vi "Sensors_DAQ.vi"() -> ()   [LabVIEW 2018]
uses:
  <vilib>/DAQmx/read.llb/DAQmx Read (Analog 1D Wfm NChan 1Samp).vi
  <vilib>/DAQmx/read.llb/DAQmx Read (Analog 1D Wfm NChan NSamp).vi
  <vilib>/DAQmx/miscellaneous.llb/DAQmx Fill In Error Info.vi
  Global.vi
panel:
  in  "Projects":string[](array[string])
  in  "Independent?":bool=TRUE
  out "file path 2":path=path "C:/Users/aspit/Git/MHDLab/Test Data/2018-06-02/H2TC/Temp Dependence/TestVI_Sensors_200C.tdms"
  in  "File Information":T1={"Project"=0, "SubFolder"="Temp Dependence", "Filename (Meas. Description)"="200C", "Measurement number"=0}
  out "tdms error":errorcluster
  out "tdms file":refnum<k34>
  out "VI name":string="Sensors_DAQ"
  in  "File Close Action":enum16{"Prompt", "Keep", "Archive", "Trash"}(ring)
  out "SD- W-F":dbl format="%#_3g"
  out "output cluster":T2={"Dynamic Data"=[{"t0"=timestamp(3609182358.6509175 s since 1904-01-01), "dt"=0.001, "Y"=[16.023829850338394, 14.80731437156387, 15.375021577144786, 15.302030648970707, 14.993846735687534, 15.172269000155545, 15.41557209302001, 14.766763858065836, 14.742433550042655, 15.39124178347577, 13.550248525884811, 15.058727558775551, 14.539680985385544, 13.801661683060253, 15.123608382269047, 14.418029448475409, 12.674357572804048, 15.07494776461089, 14.8884153990331, 14.839754782475815, 15.350691267696128, 15.001956838551372, 14.685662831542366, 15.585884261437762, 15.504783228506689, 16.486105770120822, 14.466690063070182, 15.399351886650813, 15.788636846565048, 14.937076015817745, 15.066837661690066, 15.666985295008281, 13.615129340071363, 15.050617455867389, 14.774873960752835, 13.834102090870779, 14.718103242076175, 13.939533416940243, 14.734323447380866, 14.928965913004511, 14.48291026798524, 15.934618710339358, 15.31014075207569, 14.450469858180192, 16.210362236493587, 15.545333744892353, 14.831644679738353, 15.65076508824297, 15.050617455867389, 15.107388176357638, 16.169811717473685, 14.953296221463212, 15.480452918751944, 15.285810442779812, 14.750543652710753, 14.734323447380866, 15.861627778191966, 14.328818322303867, 15.139828588205837, 14.718103242076175, 12.925770709450994, 15.293920545872076, 14.126065765635374, 13.73678086773647, 13.85843239679376, 14.945186118637316, 15.18848920616849, 15.521003435041784, 15.123608382269047, 16.23469254798311, 15.099278073411448, 14.945186118637316, 16.899721084651695, 15.302030648970707, 15.375021577144786, 15.885958088849911, 14.791094166145733, 14.969516427133946, 15.35880137083931, 13.898982906789428, 14.823534577007216, 15.602104468100684, 13.550248525884811, 14.961406324295417, 14.872195193488743, 14.158506174440262, 14.750543652710753, 14.685662831542366, 14.263937503745375, 14.815424474282388, 13.371826288905389, 13.801661683060253, 15.285810442779812, 14.336928424651816, 14.912745707396986, 15.139828588205837, 14.13417586782726, 15.602104468100684, 14.831644679738353, 14.353148629366466], "attributes"=variant("NI_ChannelName"=variant(string "CCP"), "NI_UnitDescription"=variant(string "psi"))}, {"t0"=timestamp(3609182358.6509314 s since 1904-01-01), "dt"=0.001, "Y"=[-0.027309685282801026, -0.026841327845251103, -0.028501867826300153, -0.027394841179941835, -0.02648651160096805, -0.02752257502531117, -0.029651472388779833, -0.02814705159680342, -0.02774965741606923, -0.027806428013557434, -0.029935325362275604, -0.027721272117294977, -0.029268270871504035, -0.027664501519686108, -0.02806189570126181, -0.026940676393074924, -0.027905776558968566, -0.026174273303327916, -0.02922569292492208, -0.027054217590280864, -0.027692886818500607, -0.02736645588091518, -0.029750820929721714, -0.026784557246381853, -0.030503031303541837, -0.026656823398625497, -0.02929665616920104, -0.02637297040211648, -0.028558638422732333, -0.025677530551885368, -0.029963710659519777, -0.025975576203519556, -0.029396004710987786, -0.025067246591287215, -0.029694050334926628, -0.026585860149691824, -0.029935325362275604, -0.027394841179941835, -0.02918311497829639, -0.02841671193150358, -0.027820620662916927, -0.02726710733416212, -0.02973662828103015, -0.026699401347923896, -0.03026175627943198, -0.028246400141375298, -0.03078688427133773, -0.026912291093722306, -0.029268270871504035, -0.027096795539148823, -0.02963727974005461, -0.027025832291010035, -0.02942439000859754, -0.026912291093722306, -0.02918311497829639, -0.026216851253154018, -0.030346912170450463, -0.02696906169240708, -0.030361104818936967, -0.027494189726375615, -0.0302475636309123, -0.02811866629830949, -0.029552123847602085, -0.026798749896106866, -0.029566316496356222, -0.027678694169095873, -0.029254078222648243, -0.02796254715623612, -0.02994951801090008, -0.026358777752236745, -0.03007725184830544, -0.026756171946916422, -0.03009144449688219, -0.026926483743401168, -0.030176600388242665, -0.02647231895112971, -0.029112151733822894, -0.026245236553012107, -0.029878554767729867, -0.026727786647430446, -0.030190793036786095, -0.02791996920829297, -0.029523738550079337, -0.026827135195541495, -0.02973662828103015, -0.026983254342065492, -0.029963710659519777, -0.029268270871504035, -0.030006288605350193, -0.02648651160096805, -0.02906957378708032, -0.028473482528054414, -0.030346912170450463, -0.02723872203504412, -0.030332719521959234, -0.027309685282801026, -0.030673343084445033, -0.02723872203504412, -0.028700564913467494, -0.026699401347923896], "attributes"=variant("NI_ChannelName"=variant(string "PN"), "NI_UnitDescription"=variant(string "lpm"))}], "Dynamic Data"=[{"t0"=timestamp(3609182358.7509174 s since 1904-01-01), "dt"=0.001, "Y"=[14.912259126500649], "attributes"=variant("NI_ChannelName"=variant(string "CCP (Arith. Mean)"), "NI_OriginalChannelName"=variant(string "CCP"), "NI_UnitDescription"=variant(string "psi"))}, {"t0"=timestamp(3609182358.7509317 s since 1904-01-01), "dt"=0.001, "Y"=[-0.02826243780954195], "attributes"=variant("NI_ChannelName"=variant(string "PN (Arith. Mean)"), "NI_OriginalChannelName"=variant(string "PN"), "NI_UnitDescription"=variant(string "lpm"))}], "Dynamic Data"=[], "Dynamic Data Type"=[]}
  out "file size TDMS":dbl=297.068359375
  in  "Save Data TDMS":bool=TRUE
  out "Total Heat input":dbl[unit](knob)
  out "Heat loss to water":dbl[unit](knob)
  out "SD-C-P":dbl=0.7295631112135156 format="%#_3g"
  out "SD- PNP":dbl=0.001443410184956393 format="%#_3g"
  out "Chamber Pressure":dbl[unit](knob)=102816.41626294405 scale format="%#_4g"
  out "PNP":dbl[unit](knob)=-194.86266606428845 scale format="%#_4g"
  out "Fuel Flow":dbl(knob) scale format="%#_4g"
  out "Water Flow":dbl(knob) scale format="%#_4g"
  out "SD- F-F":dbl format="%#_3g"
  in  "stop":bool
  in  "Tab Control":enum32{"File", "Setup"}(tab)=enum."Setup"
  in  "task/channels in":refnum<k21>="AllCurrents"
  in  "# HVOF":i32=4
  in  "Minimum time between \nreadings [ms]":u32=100
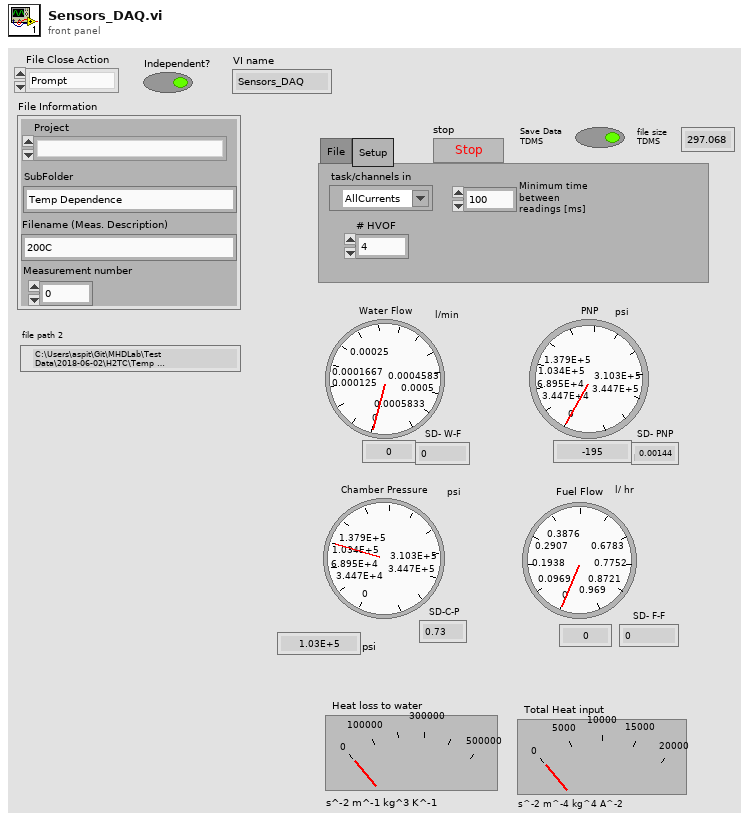
[diagram p1: front panel]
types:
  T1 = cluster{"Project":u16, "SubFolder":string, "Filename (Meas. Description)":string, "Measurement number":i32}
  T2 = cluster{"Dynamic Data":dynamicdata, "Dynamic Data":dynamicdata, "Dynamic Data":dynamicdata, "Dynamic Data Type":dynamicdata}
  T3 = cluster{waveform(dbl)[], "Arithmetic Mean":dynamicdata, waveform(dbl)[], "Arithmetic Mean":dynamicdata}
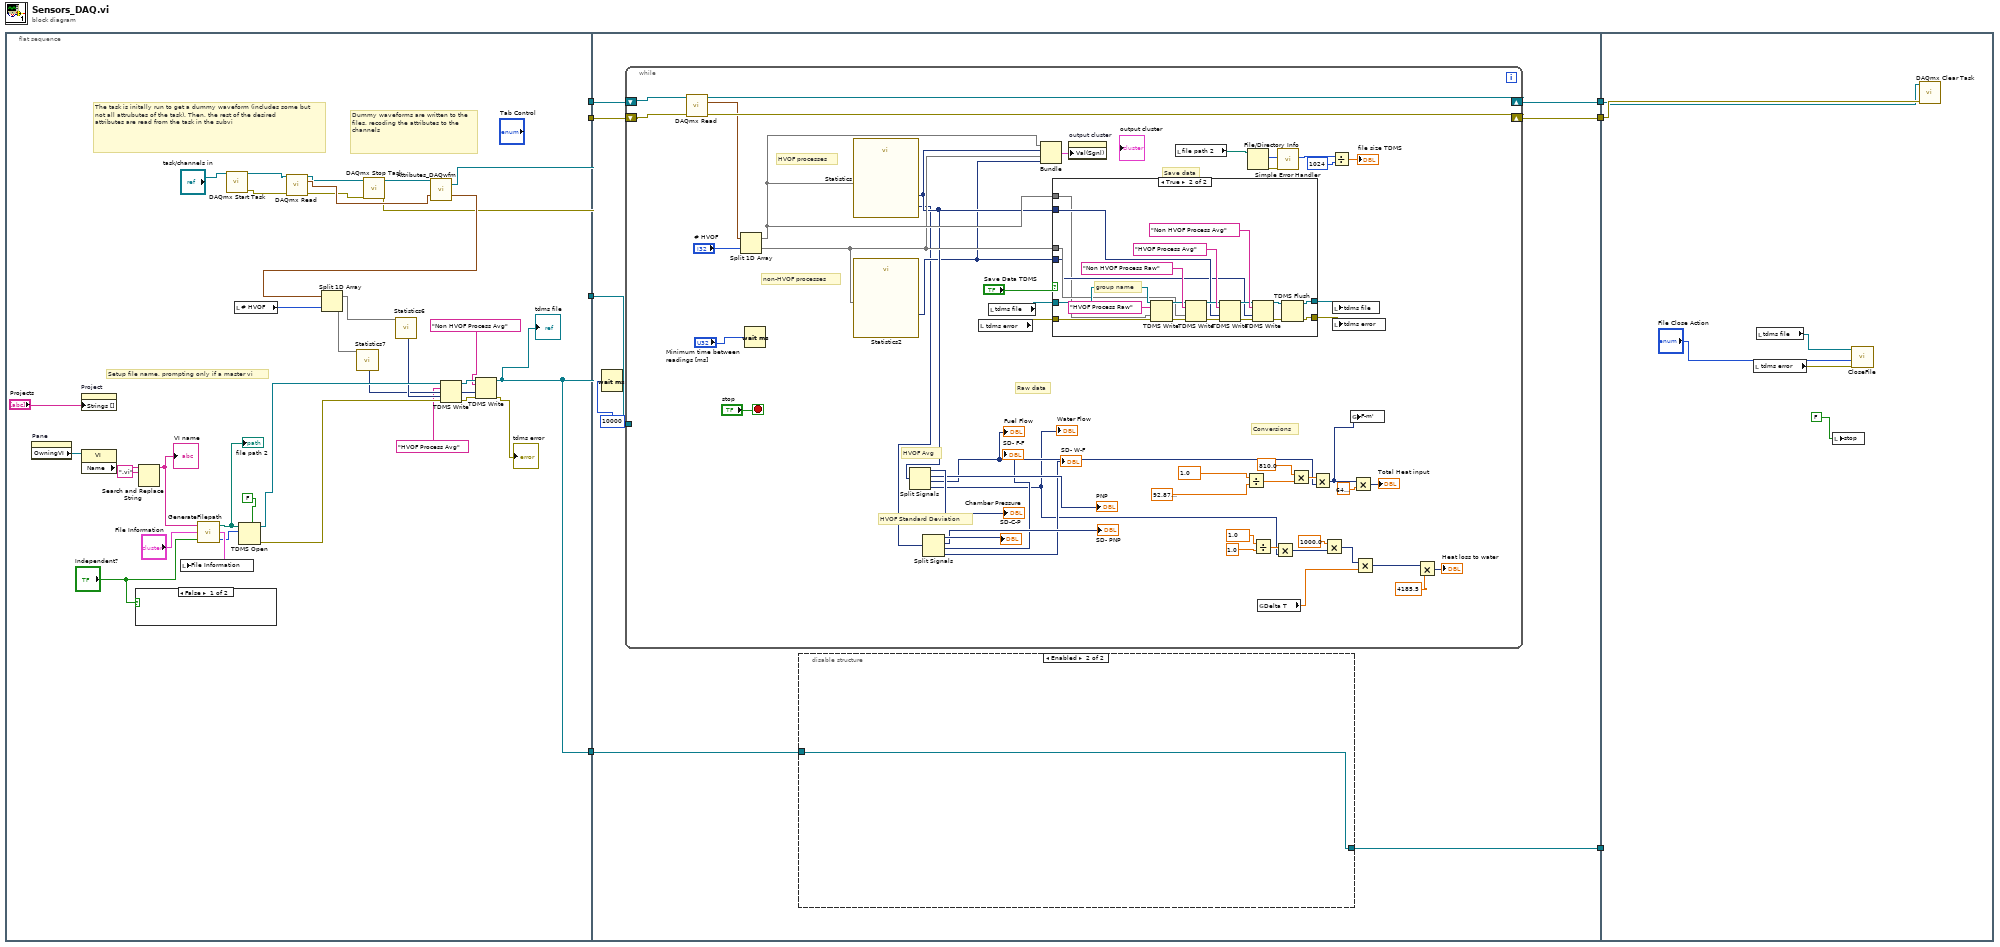
[diagram p0: block diagram]
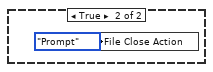
[diagram p2: hidden frame]
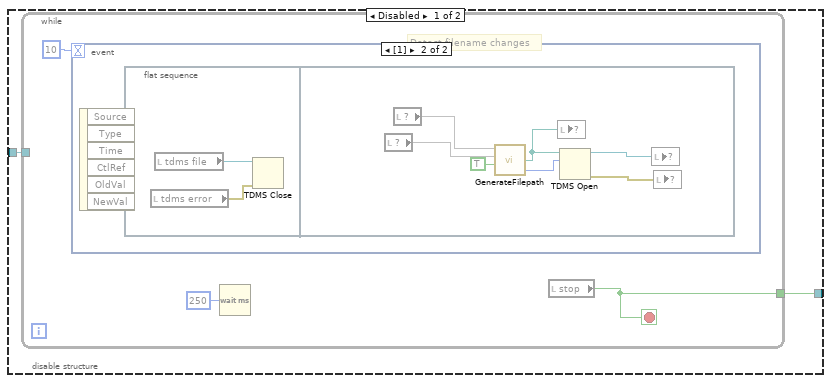
[diagram p3: hidden frame]
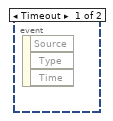
[diagram p4: hidden frame]
diagram:
  n1 = flat-sequence {
    tunnel: [w10] -> w4
    tunnel: [w8] -> w3
    tunnel: [w9] -> w2
    tunnel: [w8] -> w1
    tunnel: [w50] -> w7
    tunnel: [w48] -> w6
    tunnel: [w44] -> w5
    tunnel: w4 -> [w49]
    tunnel: w3 -> [w47]
    tunnel: w2 -> [w46]
    tunnel: w1 -> [w45]
    tunnel: w7 -> [w143]
    tunnel: w6 -> [w138]
    tunnel: w5 -> [_]
    frame #0 {
      # "Setup file name, prompting only if a master vi"
      # "Dummy waveforms are written to the files, recoding the attributes to the channels"
      # "The task is initally run to get a dummy waveform (includes some but not all attrubutes of the task). Then, the rest of the desired attributes are read from the task in the subvi"
      n2 = property on="Pane" class="Pane"() -> ("OwningVI"=w31:refnum<vi>)  [unwired: 2 in, 2 out]
      n3 = property on="Project" class="Ring (strict)"("Strings []"="Projects") -> ()  [unwired: 2 in, 2 out]
      n4 = property class="VI"(reference=w31) -> ("Name"=w30:string)  [unwired: 1 in, 2 out]
      n5 = case shown="False" "Independent?" {
        frame False {
        }
        frame True {
          n6 = local write "File Close Action"(enum16{"Prompt", "Keep", "Archive", "Trash"}."Prompt" ("File Close Action")) -> ()
        }
      }
      n7 = Search and Replace String(input string=w30, search string=".vi") -> (result string=w35:string)  [unwired: 6 in, 3 out]
      "VI name" <- w35
      n8 = call "GenerateFilepath.vi"("Check for file?"="Independent?", "File Information"="File Information", "Instrument"=w35) -> ("File Action"=w32:i32, "File Information Out"=w33:T1, "File Path Out"=w36:path)
      "file path 2" <- w36
      n9 = local write "File Information"(w33) -> ()
      n10 = call <vilib>:"DAQmx Start Task.vi"("task/channels in"="task/channels in") -> ("task out"=w16:refnum<k21>, "error out"=w17:errorcluster)  [unwired: 13 in]
      n11 = local read "# HVOF"() -> (w26:i32)
      n12 = TDMS Open(5:FALSE ("create index file? (T)"), 10:w32, 11:w36) -> (0:w40:errorcluster, 3:w39:refnum<k34>)  [unwired: 4 in]
      n13 = call-poly <vilib>:"DAQmx Read.vi"("task/channels in"=w16, "error in"=w17) -> ("task out"=w18:refnum<k21>, "data"=w21:waveform(dbl)[], "error out"=w19:errorcluster)  [unwired: 11 in]
      n14 = call <vilib>:"DAQmx Stop Task.vi"("task/channels in"=w18, "error in"=w19) -> ("task out"=w20:refnum<k21>, "error out"=w9:errorcluster)  [unwired: 12 in]
      n15 = call "Attributes_DAQwfm.vi"("data"=w21, "Refnum in"=w20) -> ("Array"=w27:waveform(dbl)[], "Refnum in 2"=w10:refnum<k21>)
      n16 = Split 1D Array(array=w27, index=w26) -> (first subarray=w25:waveform(dbl)[], second subarray=w23:waveform(dbl)[])
      n17 = call "Statistics7"("Signals"=w23) -> ("Arithmetic Mean"=w22:dynamicdata)  [unwired: 24 in, 2 out]
      n18 = call "Statistics6"("Signals"=w25) -> ("Arithmetic Mean"=w24:dynamicdata)  [unwired: 24 in, 2 out]
      n19 = TDMS Write(0:w39, 5:"HVOF Process Avg" ("group name in (Untitled)"), 9:w24, 11:w40) -> (4:w28:refnum<k34>, 15:w29:errorcluster)  [unwired: 2 in, 2 out]
      n20 = TDMS Write(0:w28, 5:"Non HVOF Process Avg" ("group name in (Untitled)"), 9:w22, 11:w29) -> (4:w8:refnum<k34>, 15:→"tdms error":errorcluster)  [unwired: 2 in, 2 out]
      "tdms file" <- w8
    }
    frame #1 {
      n21 = Wait (ms)(milliseconds to wait=10000) -> ()  [unwired: 1 out]
      n22 = while {
        shift-right: [w115] -> w50
        shift-left: w46 -> [w111]
        tunnel: w47 -> [_]
        shift-right: [w112] -> w48
        shift-left: w49 -> [w113]
        stop <- "stop" stop-if-true
        # "HVOF Standard Deviation"
        # "HVOF Avg"
        # "Save data"
        # "non-HVOF processes"
        # "HVOF processes"
        # "Conversions"
        # "Raw data"
        n23 = call-poly <vilib>:"DAQmx Read.vi"("task/channels in"=w113, "error in"=w111) -> ("task out"=w112:refnum<k21>, "data"=w83:waveform(dbl)[], "error out"=w115:errorcluster)  [unwired: 11 in]
        n24 = Split 1D Array(array=w83, index="# HVOF") -> (first subarray=w81:waveform(dbl)[], second subarray=w71:waveform(dbl)[])
        n25 = Wait (ms)(milliseconds to wait="Minimum time between \nreadings [ms]") -> ()  [unwired: 1 out]
        n26 = call "Statistics"("Signals"=w81) -> ("Standard Dev"=w67:dynamicdata, "Arithmetic Mean"=w69:dynamicdata)  [unwired: 24 in, 1 out]
        n27 = call "Statistics2"("Signals"=w71) -> ("Arithmetic Mean"=w68:dynamicdata)  [unwired: 24 in, 2 out]
        n28 = Split Signals(w69) -> (→"Chamber Pressure":dynamicdata, →"PNP":dynamicdata, w88:dynamicdata, w87:dynamicdata)  [unwired: 4 in]
        "Water Flow" <- w87
        "Fuel Flow" <- w88
        n29 = Split Signals(w67) -> (→"SD-C-P":dynamicdata, →"SD- PNP":dynamicdata, →"SD- F-F":dynamicdata, →"SD- W-F":dynamicdata)  [unwired: 4 in]
        n30 = local read "tdms error"() -> (w77:errorcluster)
        n31 = local read "tdms file"() -> (w76:refnum<k34>)
        n32 = Bundle(w81, "Arithmetic Mean"=w69, w71, "Arithmetic Mean"=w68) -> (w70:T3)  [unwired: 1 in]
        n33 = case shown="True" "Save Data TDMS" {
          tunnel: w76 -> [w117 w131]
          tunnel: w77 -> [w116 w127]
          tunnel: [w117 w137] -> w73
          tunnel: [w116 w136] -> w72
          tunnel: w69 -> [_ w120]
          tunnel: w71 -> [_ w121]
          tunnel: w68 -> [_ w119]
          tunnel: w81 -> [_ w118]
          frame False {
          }
          frame True {
            # "group name"
            n34 = TDMS Write(0:w131, 5:"HVOF Process Raw" ("group name in (Untitled)"), 9:w118, 11:w127) -> (4:w130:refnum<k34>, 15:w126:errorcluster)  [unwired: 2 in, 2 out]
            n35 = TDMS Write(0:w130, 5:"Non HVOF Process Raw" ("group name in (Untitled)"), 9:w121, 11:w126) -> (4:w129:refnum<k34>, 15:w125:errorcluster)  [unwired: 2 in, 2 out]
            n36 = TDMS Write(0:w129, 5:"HVOF Process Avg" ("group name in (Untitled)"), 9:w120, 11:w125) -> (4:w128:refnum<k34>, 15:w124:errorcluster)  [unwired: 2 in, 2 out]
            n37 = TDMS Write(0:w128, 5:"Non HVOF Process Avg" ("group name in (Untitled)"), 9:w119, 11:w124) -> (4:w123:refnum<k34>, 15:w122:errorcluster)  [unwired: 2 in, 2 out]
            n38 = TDMS Flush(4:w122, 7:w123) -> (0:w136:errorcluster, 3:w137:refnum<k34>)
          }
        }
        n39 = property on="output cluster" class="Clust (strict)"("Val(Sgnl)"=w70) -> ()  [unwired: 2 in, 2 out]
        n40 = local read "file path 2"() -> (w66:path)
        n41 = Divide(x=dbl[unit] 1.0, y=dbl[unit] 92.87999999999998) -> (x/y=w92:dbl[unit])
        n42 = File/Directory Info(path=w66) -> (size=w80:i64, error out=w78:errorcluster)  [unwired: 1 in, 5 out]
        n43 = Divide(x=dbl[unit] 1.0, y=dbl[unit] 1.0) -> (x/y=w102:dbl)
        n44 = global read "Global.vi" "Delta T"() -> (w85:dbl)
        n45 = Multiply(x=w102, y=w87) -> (x*y=w89:dynamicdata)
        n46 = call <vilib>:"Simple Error Handler.vi"("error in (no error)"=w78) -> ()  [unwired: 1 in, 8 out]
        n47 = Multiply(x=dbl[unit] 810.0 ("Rhol-F"), y=w92) -> (x*y=w94:dbl[unit])
        n48 = Multiply(x=w94, y=w88) -> (x*y=w86:dynamicdata)
        n49 = Multiply(x=dbl[unit] 1000.0 ("y"), y=w89) -> (x*y=w99:dynamicdata)
        n50 = Divide(x=w80, y=i64 1024) -> (x/y=→"file size TDMS":dbl)
        n51 = local write "tdms file"(w73) -> ()
        n52 = local write "tdms error"(w72) -> ()
        n53 = global write "Global.vi" "F-m'"(w86) -> ()
        n54 = Multiply(x=w86, y=dbl[unit] 64000000.0) -> (x*y=→"Total Heat input":dynamicdata)
        n55 = Multiply(x=w99, y=w85) -> (x*y=w100:dynamicdata)
        n56 = Multiply(x=w100, y=dbl[unit] 4185.5) -> (x*y=→"Heat loss to water":dynamicdata)
      }
      n57 = disable-structure shown="Enabled" {
        disable-tunnel: w45 -> [w52 w65]
        disable-tunnel: [w51 w65] -> w44
        frame Disabled {
          # "Detect filename changes"
          n58 = while {
            tunnel: w52 -> [_]
            tunnel: [w53] -> w51
            stop <- w53 stop-if-true
            n59 = event shown="[1]" {
              selector: _ -> [_ _]
              dyn-events: _ -> [_ _]
              timeout: 10 -> [_ _]
              event Timeout {
                n60 = event-data() -> ()  [unwired: 1 in, 3 out]
              }
              event #1 (no event record) {
                n61 = event-data() -> ()  [unwired: 1 in, 6 out]
                n62 = flat-sequence {
                  frame #0 {
                    n63 = local read "tdms error"() -> (w57:errorcluster)
                    n64 = local read "tdms file"() -> (w56:refnum<k34>)
                    n65 = TDMS Close(8:w57, 11:w56) -> ()  [unwired: 2 out]
                  }
                  frame #1 {
                    n66 = local read item#-1() -> (w64)
                    n67 = local read item#-1() -> (w63)
                    n68 = call "GenerateFilepath.vi"("Auto Date folder"=TRUE, "Filename"=w64, "base path"=w63) -> ("Numeric"=w60:i32, "file path"=w62:path)  [unwired: 1 in, 1 out]
                    n69 = local write item#-1(w62) -> ()
                    n70 = TDMS Open(10:w60, 11:w62) -> (0:w58:errorcluster, 3:w59:refnum<k34>)  [unwired: 5 in]
                    n71 = local write item#-1(w59) -> ()
                    n72 = local write item#-1(w58) -> ()
                  }
                }
              }
            }
            n73 = Wait (ms)(milliseconds to wait=u32 250) -> ()  [unwired: 1 out]
            n74 = local read "stop"() -> (w53:bool)
          }
        }
        frame Enabled {
        }
      }
    }
    frame #2 {
      n75 = local read "tdms error"() -> (w139:errorcluster)
      n76 = local read "tdms file"() -> (w140:refnum<k34>)
      n77 = local write "stop"(FALSE ("stop")) -> ()
      n78 = call "CloseFile.vi"("error in (no error)"=w139, "Action"="File Close Action", "Refnum in"=w140) -> ()  [unwired: 8 in, 1 out]
      n79 = call <vilib>:"DAQmx Clear Task.vi"("task in"=w138, "error in"=w143) -> ()  [unwired: 13 in, 1 out]
    }
  }
